vi "Register to Value.vi"(9 "Register Values":u16[](array[numeric]), 10 "Config":T1={"Config"={"Label"="", "Prefix"=0, "Address"=0, "Datatype"="", "Register Count"=0, "Multiplier"=1.0, "Offset"=0.0, "Unit"="", "Endianness"=enum."Big-Endian", "Access"=enum."R/W", "LUT"=[], "Poll Rate(ms)"=0, "Mapping"={"Module"="", "Channel"=""}}, "Custom Datatype"=refnum}, 11 "Corvus Byte Datatype in":refnum<class "Corvus Byte Datatype.lvclass">) -> (0 "Enum Value(s)":string[](array[string]), 1 "Scaled Value(s)":dbl[](array[numeric]), 2 "Ch Label(s)":string[](array[string]), 3 "Corvus Byte Datatype out":refnum<class "Corvus Byte Datatype.lvclass">)   [LabVIEW 2021, in "Corvus Byte Datatype.lvclass"]
uses:
  Corvus Byte Datatype.lvclass
  <userlib>/S2 Labs/Modbus Toolkit/TypeDefs/Config Map Type.ctl
  <userlib>/S2 Labs/Modbus Toolkit/Custom Datatype/Custom Datatype.lvclass
  <userlib>/S2 Labs/Modbus Toolkit/TypeDefs/MB Element.ctl
  <userlib>/S2 Labs/Modbus Toolkit/TypeDefs/Endianness Type.ctl
  <userlib>/S2 Labs/Modbus Toolkit/TypeDefs/Access Type.ctl
  Corvus Byte Datatype.lvclass/Corvus Byte Datatype.ctl
  <userlib>/S2 Labs/Modbus Toolkit/S2L Modbus API.lvclass
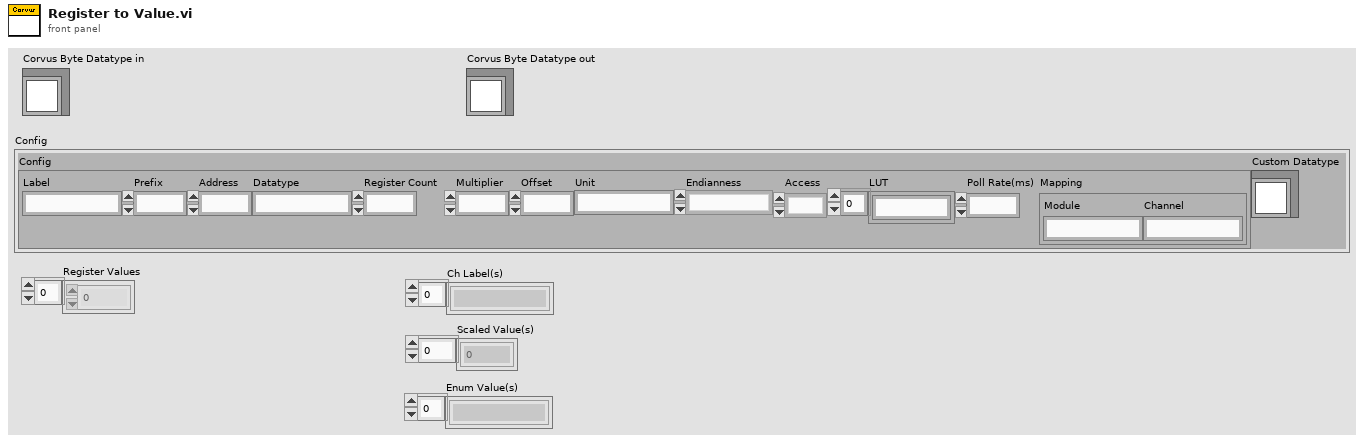
[diagram p1: front panel]
types:
  T1 = typedef "S2L Modbus API.lvclass/Config Map Type.ctl" = cluster{"Config":T2, "Custom Datatype":refnum<class "Custom Datatype.lvclass">}
  T2 = typedef "S2L Modbus API.lvclass/MB Element.ctl" = cluster{"Label":string, "Prefix":u8, "Address":u16, "Datatype":string, "Register Count":u8, "Multiplier":dbl, "Offset":dbl, "Unit":string, "Endianness":T3, "Access":T4, "LUT":string[], "Poll Rate(ms)":u16, "Mapping":cluster{"Module":string, "Channel":string}}
  T3 = typedef "Endianness Type.ctl" = enum16{"Big-Endian", "Little-Endian", "Big-Endian Byte Swap", "Little-Endian Byte Swap"}
  T4 = typedef "S2L Modbus API.lvclass/Access Type.ctl" = enum16{"R/W", "R", "W"}
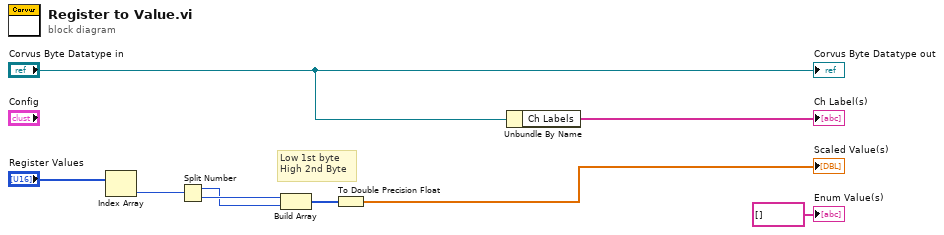
[diagram p0: block diagram]
diagram:
  # "Low 1st byte\nHigh 2nd Byte"
  n1 = Index Array(array="Register Values") -> (element=w8:u16)  [unwired: 1 in]
  n2 = Split Number(x=w8) -> (hi(x)=w6:u8, lo(x)=w7:u8)
  n3 = Build Array(w7, w6) -> (w5:u8[])
  n4 = To Double Precision Float(number=w5) -> (double precision float=→"Scaled Value(s)":dbl[])
  n5 = Unbundle By Name("Corvus Byte Datatype in") -> ("Ch Labels"=→"Ch Label(s)":string[])
  "Corvus Byte Datatype out" <- "Corvus Byte Datatype in"
  "Enum Value(s)" <- string[] [] ("Enum Value(s)")
